vi "Terminal_Control.vi"(8 "Error In":errorcluster, 10 "Text to add":string, 11 "LstBox Refnum":refnum<vi>) -> (0 "Error Out":errorcluster)   [LabVIEW 2012]
uses:
  <vilib>/Utility/error.llb/DialogType.ctl
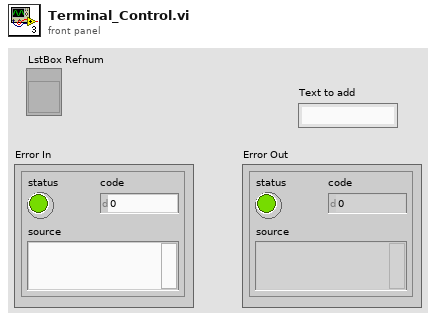
[diagram p1: front panel]
types:
  T1 = typedef "DialogType.ctl" = u16
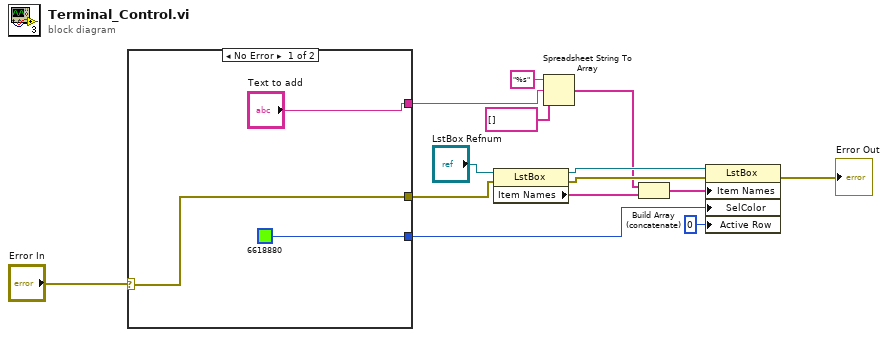
[diagram p0: block diagram]
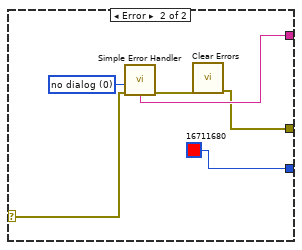
[diagram p2: hidden frame]
diagram:
  n1 = case shown="No Error" "Error In" {
    selector: "Error In" -> [w16 w20]
    tunnel: [u32 6618880 u32 16711680] -> w8
    tunnel: [w16 w19] -> w6
    tunnel: ["Text to add" w22] -> w3
    frame No Error {
    }
    frame Error {
      w21 = T1 0 items=["no dialog", "OK message", "continue or stop message", "OK message + warnings", "continue/stop + warnings"] ("type of dialog (OK msg:1)")
      n2 = call <vilib>:"Simple Error Handler.vi"("type of dialog (OK msg:1)"=w21, "error in (no error)"=w20) -> ("error out"=w23:errorcluster, "message"=w22:string)  [unwired: 3 in, 3 out]
      n3 = call <vilib>:"Clear Errors.vi"("error in (no error)"=w23) -> ("error out"=w19:errorcluster)  [unwired: 6 in]
    }
  }
  n4 = property class="LstBox"(reference="LstBox Refnum", error in=w6) -> (reference out=w11:refnum<vi>, error out=w12:errorcluster, "Item Names"=w9:string[])
  n5 = Spreadsheet String To Array(format string="%s", spreadsheet string=w3, array type (2D Dbl)=string[] []) -> (array=w2:string[])  [unwired: 1 in]
  n6 = Build Array (concatenate)(w2, w9) -> (w10:string[])
  n7 = property class="LstBox"(reference=w11, error in=w12, "Item Names"=w10, "SelColor"=w8, "Active Row"=0 ("Active Row:Active Row Number")) -> (error out=→"Error Out":errorcluster)  [unwired: 1 out]
